vi "expand int for MUX80 config.vi"(7 "RegEx":string, 8 "Input Config Str":string, 9 "Default Config Str":string, 11 "NumChannels":i32) -> (0 "Good Initial Arr":bool, 2 "Output Config Arr":i32[](array[numeric]))   [LabVIEW 2020]
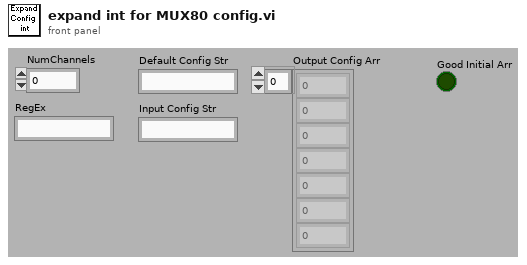
[diagram p1: front panel]
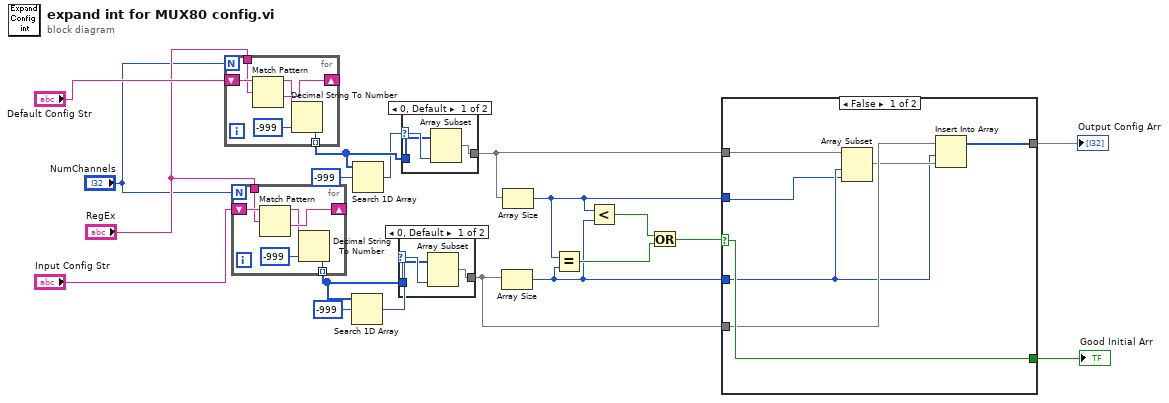
[diagram p0: block diagram]
diagram:
  n1 = for {
    N: "NumChannels" -> [_]
    shift-right: [w23] -> _
    shift-left: "Default Config Str" -> [w25]
    tunnel: "RegEx" -> [w24]
    tunnel: [w21] -> w4 mode=indexing
    n2 = Match Pattern(string=w25, regular expression=w24) -> (before substring=w22:string, after substring=w23:string)  [unwired: 1 in, 2 out]
    n3 = Decimal String To Number(string=w22, default (0L)=-999 ("default (0 I32)")) -> (number=w21:i32)  [unwired: 1 in, 1 out]
  }
  n4 = for {
    N: "NumChannels" -> [_]
    shift-right: [w29] -> _
    shift-left: "Input Config Str" -> [w31]
    tunnel: "RegEx" -> [w30]
    tunnel: [w27] -> w7 mode=indexing
    n5 = Match Pattern(string=w31, regular expression=w30) -> (before substring=w28:string, after substring=w29:string)  [unwired: 1 in, 2 out]
    n6 = Decimal String To Number(string=w28, default (0L)=-999 ("default (0 I32)")) -> (number=w27:i32)  [unwired: 1 in, 1 out]
  }
  n7 = Search 1D Array(1D array=w7, element=-999) -> (index of element=w8:i32)  [unwired: 1 in]
  n8 = Search 1D Array(1D array=w4, element=-999) -> (index of element=w3:i32)  [unwired: 1 in]
  n9 = case shown="0, Default" w8 {
    selector: w8 -> [w34 _]
    tunnel: [w33 w35] -> w2
    tunnel: w7 -> [w32 w35]
    frame 0, Default {
      n10 = Array Subset(array=w32, length=w34) -> (w33:i32[])  [unwired: 1 in]
    }
    frame -1 {
    }
  }
  n11 = case shown="0, Default" w3 {
    selector: w3 -> [w38 _]
    tunnel: [w37 w39] -> w5
    tunnel: w4 -> [w36 w39]
    frame 0, Default {
      n12 = Array Subset(array=w36, length=w38) -> (w37:i32[])  [unwired: 1 in]
    }
    frame -1 {
    }
  }
  n13 = Array Size(array=w2) -> (size(s)=w9:i32)
  n14 = Array Size(array=w5) -> (size(s)=w1:i32)
  n15 = Equal?(x=w1, y=w9) -> (x = y?=w17:bool)
  n16 = Less?(x=w1, y=w9) -> (x < y?=w18:bool)
  n17 = Or(x=w18, y=w17) -> (x .or. y?=w16:bool)
  n18 = case shown="False" w16 {
    selector: w16 -> [w46 w48]
    tunnel: [w46 w48] -> w19
    tunnel: w5 -> [w45 _]
    tunnel: w2 -> [w44 w47]
    tunnel: w9 -> [w41 _]
    tunnel: [w42 w47] -> w11
    tunnel: w1 -> [w40 _]
    frame False {
      n19 = Array Subset(array=w45, index=w41, length=w40) -> (w43:i32[])
      n20 = Insert Into Array(array=w44, index=w41, new element=w43) -> (w42:i32[])
    }
    frame True {
    }
  }
  "Good Initial Arr" <- w19
  "Output Config Arr" <- w11
